vi "ReceiveEth.vi"(1 "Cnt in":u32, 2 "queue out":refnum<queue>, 3 "reference":refnum<vi>) -> (0 "Cnt out":u32)   [LabVIEW 2010]
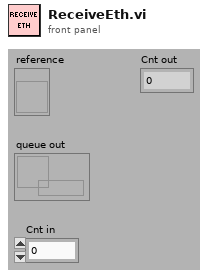
[diagram p1: front panel]
types:
  T1 = enum16{"Standard", "Buffered", "CRLF", "Immediate"}
  T2 = cluster{"ID":u32, "MSGTYPE":u8, "LEN":u8, "aDATA":u8[]}
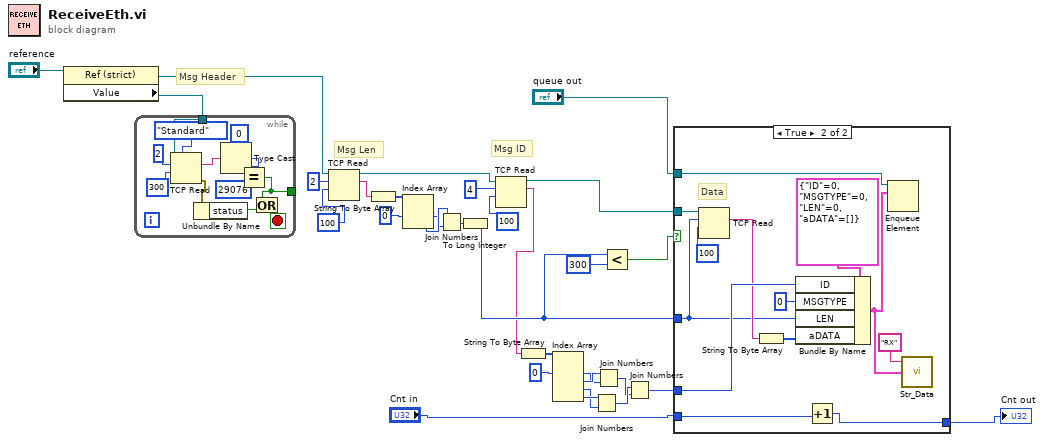
[diagram p0: block diagram]
diagram:
  # "Msg Header"
  # "Msg Len"
  # "Msg ID"
  n1 = property class="Ref (strict)"(reference="reference") -> ("Value"=w2:refnum<k5>)  [unwired: 1 in, 2 out]
  n2 = while {
    tunnel: w2 -> [w40]
    tunnel: [w36] -> _
    stop <- w37 stop-if-true
    n3 = TCP Read(connection ID=w40, bytes to read=2, 7:T1."Standard" ("mode (standard)"), 9:300) -> (data out=w34:string, error out=w39:errorcluster)  [unwired: 1 in, 1 out]
    n4 = Unbundle By Name(w39) -> ("status"=w38:bool)
    n5 = Type Cast(type=u16 0 ("y"), x=w34) -> (*(type *) &x=w32:u16)
    n6 = Equal?(x=w32, y=u16 29076) -> (x = y?=w36:bool)
    n7 = Or(x=w36, y=w38) -> (x .or. y?=w37:bool)
  }
  n8 = TCP Read(connection ID=w2, bytes to read=2, 9:100) -> (connection ID out=w6:refnum<k5>, data out=w7:string)  [unwired: 2 in, 1 out]
  n9 = String To Byte Array(string=w7) -> (unsigned byte array=w9:u8[])
  n10 = Index Array(array=w9, index #1=0 ("index")) -> (element #1=w10:u8, element #2=w11:u8)  [unwired: 1 in]
  n11 = Join Numbers(hi=w11, lo=w10) -> ((hi.lo)=w12:u16)
  n12 = To Long Integer(number=w12) -> (32bit integer=w25:i32)
  n13 = TCP Read(connection ID=w6, bytes to read=4, 9:100) -> (connection ID out=w28:refnum<k5>, data out=w16:string)  [unwired: 2 in, 1 out]
  n14 = String To Byte Array(string=w16) -> (unsigned byte array=w14:u8[])
  n15 = Index Array(array=w14, index #1=0 ("index")) -> (element #1=w17:u8, element #2=w18:u8, element #3=w19:u8, element #4=w20:u8)  [unwired: 3 in]
  n16 = Join Numbers(hi=w20, lo=w19) -> ((hi.lo)=w22:u16)
  n17 = Join Numbers(hi=w18, lo=w17) -> ((hi.lo)=w21:u16)
  n18 = Less?(x=w25, y=300) -> (x < y?=w27:bool)
  n19 = Join Numbers(hi=w22, lo=w21) -> ((hi.lo)=w23:u32)
  n20 = case shown="True" w27 {
    tunnel: "queue out" -> [_ w55]
    tunnel: "Cnt in" -> [w43 w45]
    tunnel: [w43 w44] -> w30
    tunnel: w25 -> [_ w46]
    tunnel: w23 -> [_ w50]
    tunnel: w28 -> [_ w48]
    frame False {
    }
    frame True {
      # "Data"
      n21 = TCP Read(connection ID=w48, bytes to read=w46, 9:100) -> (data out=w47:string)  [unwired: 2 in, 2 out]
      n22 = String To Byte Array(string=w47) -> (unsigned byte array=w51:u8[])
      n23 = Bundle By Name(cluster=T2 {"ID"=0, "MSGTYPE"=0, "LEN"=0, "aDATA"=[]} ("Msg"), "ID"=w50, "MSGTYPE"=u8 0, "LEN"=w46, "aDATA"=w51) -> (w53:T2)
      n24 = Increment(x=w45) -> (x+1=w44:u32)
      n25 = Enqueue Element(queue=w55, element=w53) -> ()  [unwired: 1 in, 4 out]
      n26 = call "Str_Data.vi"("Msg"=w53, "string"="RX") -> ()  [unwired: 1 in, 1 out]
    }
  }
  "Cnt out" <- w30
